vi "Method.vi"(4 "Input B":refnum<class "Abs_Numeric.lvclass">, 5 "Input A":refnum<class "Abs_Complex Extended Float.lvclass">) -> (1 "Result":T1)   [LabVIEW 2021, in "Subtract_CPLX_EXT.lvclass"]
uses:
  Subtract_CPLX_EXT.lvclass
  Abs_Types/Complex Extended Float/Abs_Complex Extended Float.lvclass
  Abs Type.ctl
  Abs_Types/Numeric/Abs_Numeric.lvclass
  C:/TSA/LV_Abstract/Source/Functions/Support/Function/Two Terminal/Cmplx EXT/AbsFunc_Two Term_Complex EXT.lvclass
  C:/Program Files (x86)/National Instruments/LabVIEW 2021/vi.lib/TSA/Abstract Data Classes/Abs_Types/Complex Extended Float/Abs_Complex Extended Float.lvclass
  Support/Function/Two Terminal/Cmplx EXT/AbsFunc_Two Term_Complex EXT.lvclass/AbsFunc_Two Term_Complex EXT.ctl
  Support/Function/Two Terminal/Cmplx EXT/Properties/Write Numeric A.vi
  Support/Function/Two Terminal/Cmplx EXT/Properties/Write Numeric B.vi
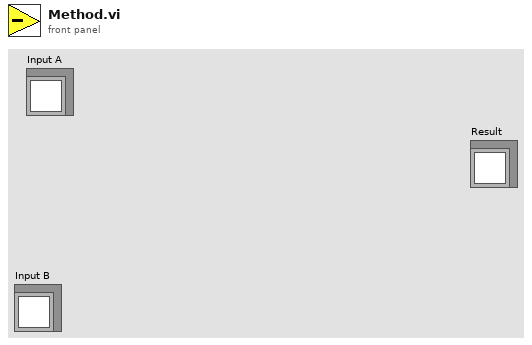
[diagram p1: front panel]
types:
  T1 = typedef "Subtract_CPLX_EXT.lvclass/Abs Type.ctl" = refnum<class "Abs_Complex Extended Float.lvclass">
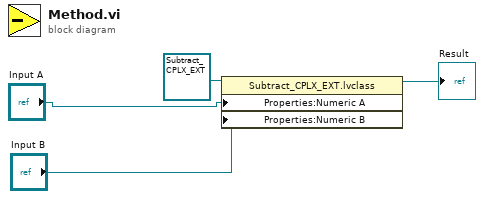
[diagram p0: block diagram]
diagram:
  n1 = property class="Subtract_CPLX_EXT.lvclass"(reference=refnum<class "Subtract_CPLX_EXT.lvclass"> refnum ("Subtract_DBL.lvclass"), "Properties:Numeric A"="Input A", "Properties:Numeric B"="Input B") -> (reference out=→"Result":refnum<class "Subtract_CPLX_EXT.lvclass">)  [unwired: 1 in, 1 out]
